vi "Gray's GUI.vi"() -> ()   [LabVIEW 2009]
uses:
  <vilib>/rvi/interface/nirviOpenFPGA/nirviOpenFPGA.xnode
  <vilib>/userDefined/High Color/nirio_resource_hc.ctl
  <vilib>/rvi/interface/nirviReadWriteControl/nirviReadWriteControl.xnode
  Athena Brain.lvproj_FPGA Target 2_Gray's Mod Motor C~4B.lvbitx
  FPGA/Gray's Mod Motor Controler.vi
  <vilib>/rvi/errors/niLvFpgaWhatHappensToTopLevelVI.ctl
  <vilib>/rvi/interface/common/niFpgaNodeNameForErrorReporting.ctl
  <vilib>/rvi/errors/niLvFpgaAdjustHostInterfaceError.vi
  <vilib>/rvi/interface/nirviCloseFPGA/nirviCloseFPGA.xnode
  <vilib>/FPGAPlugInAG/sbRIO-9642/nirviIntfClose_sbRIO-9642.vi
  <vilib>/rvi/interface/nirviMethod/nirviMethod.xnode
  Strict Lidar Motor Control Cluster.ctl
  Strict Lidar Motor Indicator Cluster.ctl
  NiRioSrv.dll
  <vilib>/Utility/error.llb/Error Cluster From Error Code.vi
  <vilib>/FPGAPlugInAG/sbRIO-9642/nirviIntfOpen_sbRIO-9642.vi
  <vilib>/RVI Host/nirviSupport.llb/nirviErrorClusterFromErrorCode.vi
  <vilib>/LabVIEW Targets/FPGA/RIO/nirio_HostInterface/nirio_WriteBig.vi
  <vilib>/Utility/error.llb/Merge Errors.vi
  <vilib>/LabVIEW Targets/FPGA/RIO/nirio_HostInterface/nirio_Reset.vi
  <vilib>/LabVIEW Targets/FPGA/RIO/nirio_HostInterface/nirio_DMAStopAll.vi
  <vilib>/LabVIEW Targets/FPGA/RIO/nirio_HostInterface/nirio_DisableInterrupts.vi
  Strict Drive Motor Control Cluster.ctl
  Strict Steering Motor Control Cluster.ctl
  Strict Raw Encoder Cluster.ctl
  Strict Steering Motor Indicator Cluster.ctl
  FPGA/Motor Control/Strict Custom Compensator.ctl
panel:
  out "Drive Encoder":i32
  out "Lidar Encoder":i32
  out "Steering Encoder":i32
  out "Drive Speed, Measured (ft/sec)":fxp<+/-,14,4> format="%.12g"
  in  "Custom Compensator":T1={"Zero coefficients"=[0.0, 0.0, 0.0, 0.0, 0.0, 0.0], "Pole coefficients"=[0.0, 0.0, 0.0, 0.0, 0.0, 0.0], "Gain"=0.0}
  out "Lidar Motor Indicator":T2
  out "Steering Motor Indicator":T3
  out "Drive Motor Indicator":T4 {"Speed (ft/sec)" format="%.12g"; "Output Voltage" format="%.17g"}
  out "Encoder Information 2":T5
  in  "Lidar Motor Control":T6={"Reset Encoder"=FALSE, "Motor Enable"=FALSE, "Choice of Control Type"=enum."Direct Voltage Control", "Choice of Oscillation"=enum."Oscillate Voltage", "Choice of Compensation"=enum."None", "Choice of Error"=enum."Gray Error", "Units of pi rad 18b (s-fxp-1)"={"Phi_B Set Point (pi rad)"=0.0, "Phi_A Set Point (pi rad)"=0.0, "Phi_Lidar Set Point (pi rad)"=0.0, "Phi_Lidar - Phi_A"=0.0, "Phi_mass-Phi_Lidar"=0.0, "Convert (enc) to (pi rad)"=0.0, "Oscillation Frequency (pi rad per 100KHz)"=0.0}, "Units of 18b (s-fxp-1) gain"={"Proportional Gain"=0.0, " Integral Gain"=0.0, "Oscillation Setpoint Amplitude"=0.0, "Gravity Compensation Gain"=0.0, "Phi_B Set Point (enc) pre-gain"=0.0, "Phi_B Set Point (pi rad) pre-gain"=0.0, "Phi_A Set Point (pi rad) pre-gain"=0.0, "Phi_Lidar Set Point (pi rad) pre-gain"=0.0, "Derivative Gain"=0.0, "Double Integral Gain"=0.0, "Second Derivative Gain"=0.0}, "Units of 20b s-fxp-5 Voltage"={"Oscillation Voltage Amplitude"=0.0, "Motor Voltage"=0.0}, "Units of encoder 32b uint"={"Phi_B Set Point (enc)"=0, "Lidar Encoder Cap"=0}, "Debug Args"=[FALSE, FALSE, FALSE, FALSE, FALSE, FALSE, FALSE, FALSE, FALSE, FALSE, FALSE, FALSE, FALSE, FALSE, FALSE, FALSE, FALSE, FALSE, FALSE, FALSE], "Units of 8b int gain exponents"={"Proportional Gain"=0, " Integral Gain"=0, "Oscillation Setpoint Amplitude"=0, "Gravity Compensation Gain"=0, "Phi_B Set Point (enc) pre-gain"=0, "Phi_B Set Point (pi rad) pre-gain"=0, "Phi_A Set Point (pi rad) pre-gain"=0, "Phi_Lidar Set Point (pi rad) pre-gain"=0, "Derivative Gain"=0, "Double Integral Gain"=0, "Second Derivative Gain"=0}} {"Units of 20b s-fxp-5 Voltage"."Motor Voltage" format="%.17g"}
  in  "Steering Motor Control":T7 {"Motor Voltage" format="%.17g"}
  in  "Drive Motor Control":T8 {"Motor Voltage" format="%.17g"}
  in  "Restart on Stop":bool
  in  "resource name":T9="RIO0"
  in  "Stop":bool=TRUE
  # "50Hz Update Frequency"
  # "50 Hz Update Frequency"
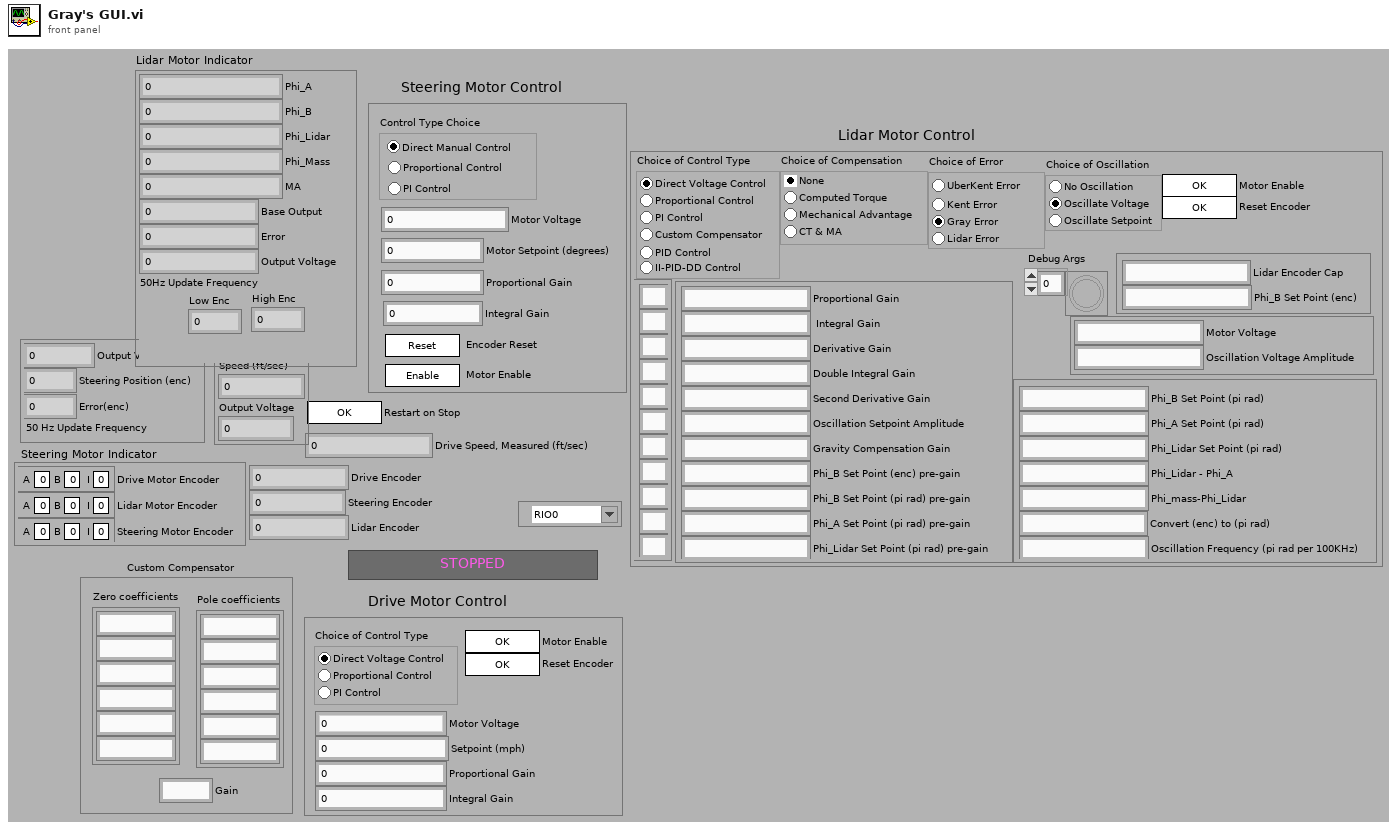
[diagram p1: front panel]
types:
  T1 = typedef "Strict Custom Compensator.ctl" = cluster{"Zero coefficients":fxp<+/-,18,1>[], "Pole coefficients":fxp<+/-,18,1>[], "Gain":fxp<+/-,18,1>}
  T2 = typedef "Strict Lidar Motor Indicator Cluster.ctl" = cluster{"Phi_A":fxp<+/-,18,1>, "Phi_B":fxp<+/-,18,1>, "Output Voltage":fxp<+/-,20,5>, "Phi_Lidar":fxp<+/-,18,1>, "Phi_Mass":fxp<+/-,18,1>, "MA":fxp<+/-,18,1>, "Base Output":fxp<+/-,18,1>, "Error":fxp<+/-,18,1>, "Low Enc":i32, "High Enc":i32}
  T3 = typedef "Strict Steering Motor Indicator Cluster.ctl" = cluster{"Output Voltage":fxp<+/-,20,5>, "Steering Position (enc)":i32, "Error(enc)":i32}
  T4 = cluster{"Speed (ft/sec)":fxp<+/-,14,4>, "Output Voltage":fxp<+/-,20,5>}
  T5 = typedef "Strict Raw Encoder Cluster.ctl" = cluster{"Drive Motor Encoder":cluster{"A":bool, "B":bool, "I":bool}, "Lidar Motor Encoder":cluster{"A":bool, "B":bool, "I":bool}, "Steering Motor Encoder":cluster{"A":bool, "B":bool, "I":bool}}
  T6 = typedef "Strict Lidar Motor Control Cluster.ctl" = cluster{"Reset Encoder":bool, "Motor Enable":bool, "Choice of Control Type":enum32{"Direct Voltage Control", "Proportional Control", "PI Control", "Custom Compensator", "PID Control", "II-PID-DD Control"}, "Choice of Oscillation":enum32{"Oscillate Voltage", "Oscillate Setpoint", "No Oscillation"}, "Choice of Compensation":enum32{"None", "Computed Torque", "Mechanical Advantage", "CT & MA "}, "Choice of Error":enum32{"Gray Error", "Lidar Error", "Kent Error", "UberKent Error"}, "Units of pi rad 18b (s-fxp-1)":cluster{"Phi_B Set Point (pi rad)":fxp<+/-,18,1>, "Phi_A Set Point (pi rad)":fxp<+/-,18,1>, "Phi_Lidar Set Point (pi rad)":fxp<+/-,18,1>, "Phi_Lidar - Phi_A":fxp<+/-,18,1>, "Phi_mass-Phi_Lidar":fxp<+/-,18,1>, "Convert (enc) to (pi rad)":fxp<+/-,18,1>, "Oscillation Frequency (pi rad per 100KHz)":fxp<+/-,18,1>}, "Units of 18b (s-fxp-1) gain":cluster{"Proportional Gain":fxp<+/-,18,1>, " Integral Gain":fxp<+/-,18,1>, "Oscillation Setpoint Amplitude":fxp<+/-,18,1>, "Gravity Compensation Gain":fxp<+/-,18,1>, "Phi_B Set Point (enc) pre-gain":fxp<+/-,18,1>, "Phi_B Set Point (pi rad) pre-gain":fxp<+/-,18,1>, "Phi_A Set Point (pi rad) pre-gain":fxp<+/-,18,1>, "Phi_Lidar Set Point (pi rad) pre-gain":fxp<+/-,18,1>, "Derivative Gain":fxp<+/-,18,1>, "Double Integral Gain":fxp<+/-,18,1>, "Second Derivative Gain":fxp<+/-,18,1>}, "Units of 20b s-fxp-5 Voltage":cluster{"Oscillation Voltage Amplitude":fxp<+/-,20,5>, "Motor Voltage":fxp<+/-,20,5>}, "Units of encoder 32b uint":cluster{"Phi_B Set Point (enc)":i32, "Lidar Encoder Cap":i32}, "Debug Args":bool[], "Units of 8b int gain exponents":cluster{"Proportional Gain":i8, " Integral Gain":i8, "Oscillation Setpoint Amplitude":i8, "Gravity Compensation Gain":i8, "Phi_B Set Point (enc) pre-gain":i8, "Phi_B Set Point (pi rad) pre-gain":i8, "Phi_A Set Point (pi rad) pre-gain":i8, "Phi_Lidar Set Point (pi rad) pre-gain":i8, "Derivative Gain":i8, "Double Integral Gain":i8, "Second Derivative Gain":i8}}
  T7 = typedef "Strict Steering Motor Control Cluster.ctl" = cluster{"Encoder Reset":bool, "Motor Voltage":fxp<+/-,20,5>, "Proportional Gain":fxp<+/-,20,5>, "Motor Setpoint (degrees)":i32, "Control Type Choice":enum32{"Direct Manual Control", "Proportional Control", "PI Control"}, "Integral Gain":fxp<+/-,20,5>, "Motor Enable":bool}
  T8 = typedef "Strict Drive Motor Control Cluster.ctl" = cluster{"Motor Voltage":fxp<+/-,20,5>, "Setpoint (mph)":fxp<+/-,20,7>, "Proportional Gain":fxp<+/-,20,5>, "Choice of Control Type":enum32{"Direct Voltage Control", "Proportional Control", "PI Control"}, "Integral Gain":fxp<+/-,20,5>, "Reset Encoder":bool, "Motor Enable":bool}
  T9 = typedef "nirio_resource_hc.ctl" = tag
  T10 = typedef "niFpgaNodeNameForErrorReporting.ctl" = enum16{"Open FPGA VI Reference", "Read/Write Control", "Invoke Method: Abort", "Invoke Method: Acknowledge IRQ", "Invoke Method: Download", "Invoke Method: FIFO.Configure", "Invoke Method: FIFO.Read", "Invoke Method: FIFO.Start", "Invoke Method: FIFO.Stop", "Invoke Method: FIFO.Write", "Invoke Method: Reset", "Invoke Method: Run", "Invoke Method: Wait on IRQ", "Close FPGA VI Reference"}
  T11 = typedef "niLvFpgaWhatHappensToTopLevelVI.ctl" = enum16{"top level VI scripted behind XNode", "top level VI inlined behind XNode"}
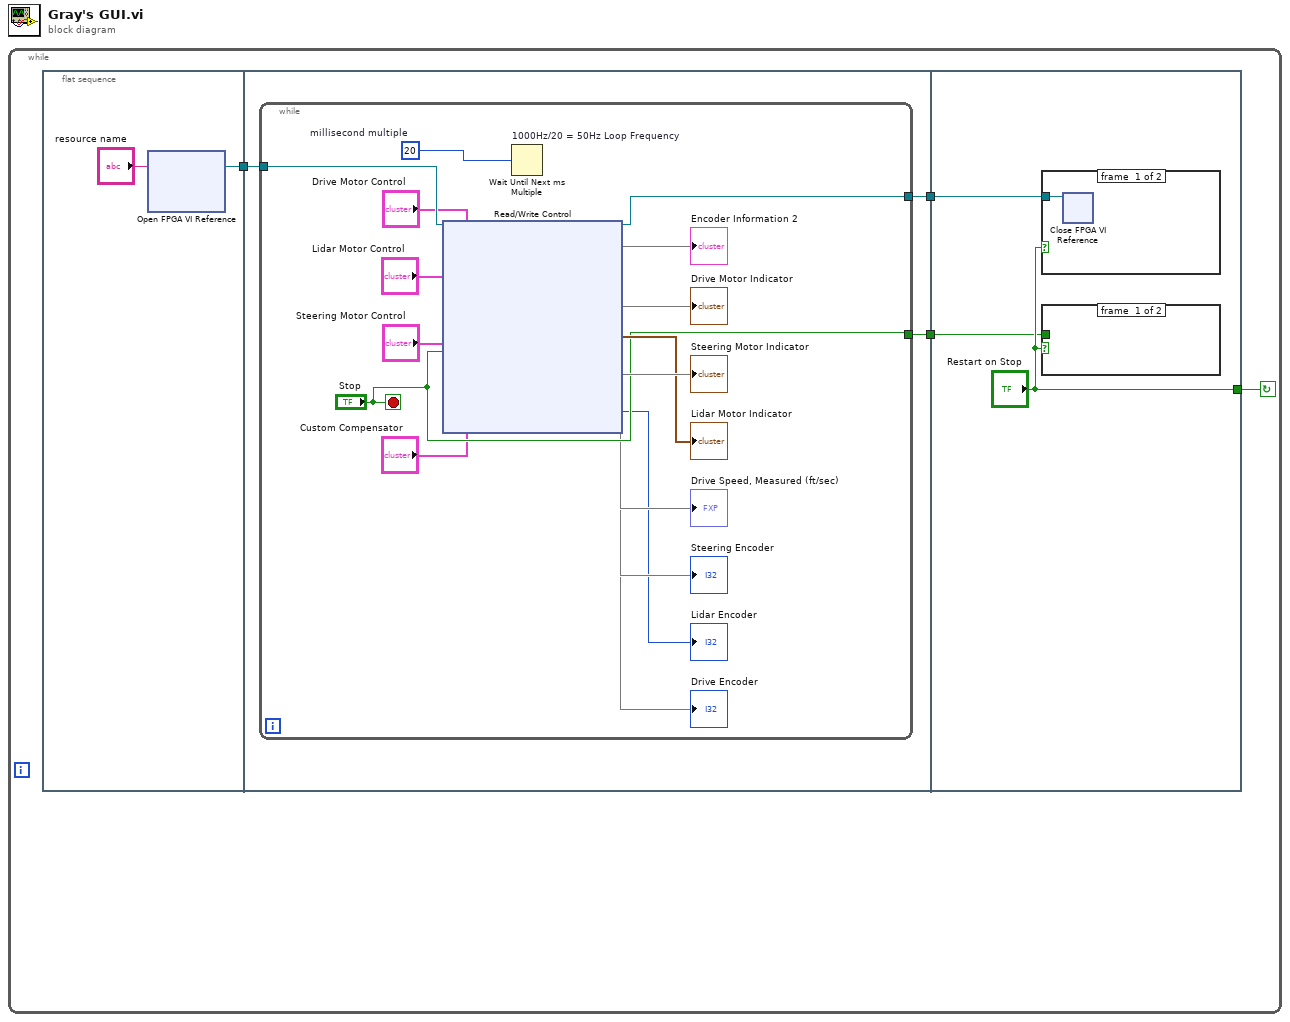
[diagram p0: block diagram]
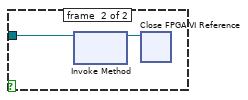
[diagram p2: hidden frame]
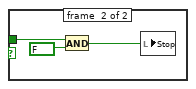
[diagram p3: hidden frame]
diagram:
  n1 = while {
    stop <- w3 continue-if-true
    n2 = flat-sequence {
      tunnel: [w5] -> w2
      tunnel: [w20] -> w4
      tunnel: w2 -> [w19]
      tunnel: [w18] -> w1
      tunnel: ["Restart on Stop"] -> w3
      tunnel: w4 -> [w155]
      tunnel: w1 -> [w154]
      frame #0 {
        n3 = xnode "Open FPGA VI Reference"("resource name"="resource name") -> ("FPGA VI Reference Out"=w5:refnum<k20>)  [unwired: 1 in, 1 out]
      }
      frame #1 {
        n4 = while {
          tunnel: ["Stop"] -> w20
          tunnel: w19 -> [w36]
          tunnel: [w35] -> w18
          stop <- "Stop" stop-if-true
          w34 = u32 20  # millisecond multiple
          n5 = xnode "Read/Write Control"("FPGA VI Reference In"=w36, "Drive Motor Control"="Drive Motor Control", "Lidar Motor Control"="Lidar Motor Control", "Steering Motor Control"="Steering Motor Control", "Stop"="Stop", "Custom Compensator"="Custom Compensator") -> ("FPGA VI Reference Out"=w35:refnum<k20>, "Encoder Information"=→"Encoder Information 2", "Drive Motor Indicator"=→"Drive Motor Indicator", "Steering Motor Indicator"=→"Steering Motor Indicator", "Lidar Motor Indicator"=→"Lidar Motor Indicator":T2, "Drive Speed, Measured (ft/sec)"=→"Drive Speed, Measured (ft/sec)", "Steering Encoder"=→"Steering Encoder", "Lidar Encoder"=→"Lidar Encoder":i32, "Drive Encoder"=→"Drive Encoder")  [unwired: 1 in, 1 out]
          n6 = Wait Until Next ms Multiple "1000Hz/20 = 50Hz Loop Frequency"(millisecond multiple=w34) -> ()  [unwired: 1 out]
        }
      }
      frame #2 {
        n7 = case shown="False" "Restart on Stop" {
          tunnel: w154 -> [w157 w167]
          frame #0 {
            n8 = xnode "Close FPGA VI Reference"("FPGA VI Reference In"=w157) -> ()  [unwired: 1 in, 1 out]
          }
          frame #1 {
            n9 = xnode "Invoke Method"("FPGA VI Reference In"=w167) -> ("FPGA VI Reference Out"=w166:refnum<k20>)  [unwired: 1 in, 1 out]
            n10 = xnode "Close FPGA VI Reference"("FPGA VI Reference In"=w166) -> ()  [unwired: 1 in, 1 out]
          }
        }
        n11 = case shown="True" "Restart on Stop" {
          tunnel: w155 -> [_ w263]
          frame #0 {
          }
          frame #1 {
            n12 = And(x=w263, y=FALSE) -> (x .and. y?=w261:bool)
            n13 = local write "Stop"(w261) -> ()
          }
        }
      }
    }
  }
